vi "GetExample.vi"(9 "# Devices":enum32{"Page 1", "Page 2", "Page 3"}(ring), 10 "Listbox":i32, 11 "ListBox in":refnum<vi>) -> (1 "image":picture, 2 "description":string, 3 "name":string, 4 "Python":string)   [LabVIEW 2019]
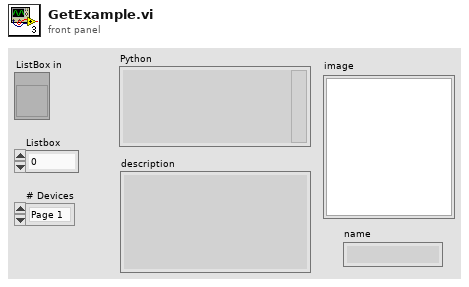
[diagram p1: front panel]
types:
  T1 = typedef "imagedata.ctl" = cluster{"image type":i32, "image depth":i32, "image":u8[], "mask":u8[], "colors":u32[], "Rectangle":cluster{"left":i16, "top":i16, "right":i16, "bottom":i16}}
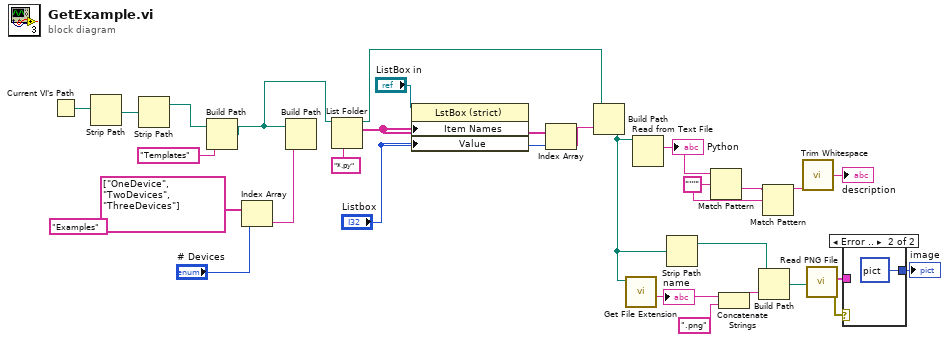
[diagram p0: block diagram]
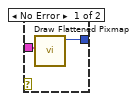
[diagram p2: hidden frame]
diagram:
  (unwired) "Examples" ("name or relative path")
  w13 = "'''" ("regular expression")
  n1 = Current VI's Path() -> (path=w23:path)
  n2 = Strip Path(path=w23) -> (stripped path=w19:path)  [unwired: 1 out]
  n3 = Strip Path(path=w19) -> (stripped path=w18:path)  [unwired: 1 out]
  n4 = Build Path(base path=w18, name or relative path="Templates") -> (appended path=w2:path)
  n5 = Index Array(array=string[] ["OneDevice", "TwoDevices", "ThreeDevices"], index="# Devices") -> (element=w28:string)
  n6 = Build Path(base path=w2, name or relative path=w28) -> ()  [unwired: 1 out]
  n7 = List Folder(path=w2, pattern="*.py") -> (path out=w16:path, filenames=w21:string[])  [unwired: 2 in, 2 out]
  n8 = property on="Property Node" class="LstBox (strict)"(reference="ListBox in", "Item Names"=w21, "Value"="Listbox") -> ()  [unwired: 1 in, 2 out]
  n9 = Index Array(array=w21, index="Listbox") -> (element=w17:string)
  n10 = Build Path(base path=w16, name or relative path=w17) -> (appended path=w8:path)
  n11 = call <vilib>:"Get File Extension.vi"("file"=w8) -> ("filename without extension"=w10:string)  [unwired: 6 in, 4 out]
  "name" <- w10
  n12 = Read from Text File(file (use dialog)=w8) -> (text=w15:string)  [unwired: 3 in, 3 out]
  "Python" <- w15
  n13 = Strip Path(path=w8) -> (stripped path=w6:path)  [unwired: 1 out]
  n14 = Match Pattern(string=w15, regular expression=w13) -> (after substring=w14:string)  [unwired: 1 in, 3 out]
  n15 = Concatenate Strings(w10, ".png" ("string")) -> (w7:string)
  n16 = Build Path(base path=w6, name or relative path=w7) -> (appended path=w5:path)
  n17 = Match Pattern(string=w14, regular expression=w13) -> (before substring=w12:string)  [unwired: 1 in, 3 out]
  n18 = call <vilib>:"Trim Whitespace.vi"("string"=w12) -> ("trimmed string"=→"description":string)  [unwired: 1 in]
  n19 = call <vilib>:"Read PNG File.vi"("path to PNG file"=w5) -> ("error out"=w1:errorcluster, "image data"=w4:T1)  [unwired: 8 in, 1 out]
  n20 = case shown="Error .." w1 {
    tunnel: w4 -> [w30 _]
    tunnel: [w29 picture data[5B] ("new picture")] -> w3
    frame No Error {
      n21 = call <vilib>:"Draw Flattened Pixmap.vi"("image data"=w30) -> ("new picture"=w29:picture)  [unwired: 8 in]
    }
    frame Error {
    }
  }
  "image" <- w3
